vi "Get Firmware Version Names.vi"(8 "Error In":errorcluster, 9 "Device ID":u8, 11 "Device Family":T1) -> (0 "Error Out":errorcluster, 2 "Firmware Version Relative Path":string[](array[string]), 3 "Firmware Version Names":string[](array[string]))   [LabVIEW 2013, in "LVH-LINX.lvlib"]
doc: "Get Firmware Version Names for user specified Device Famile and Device ID."
uses:
  <vilib>/LabVIEW Hacker/LINX/LVH-LINX.lvlib
  <vilib>/LabVIEW Hacker/LINX/Private/Type Defs/Device Family.ctl
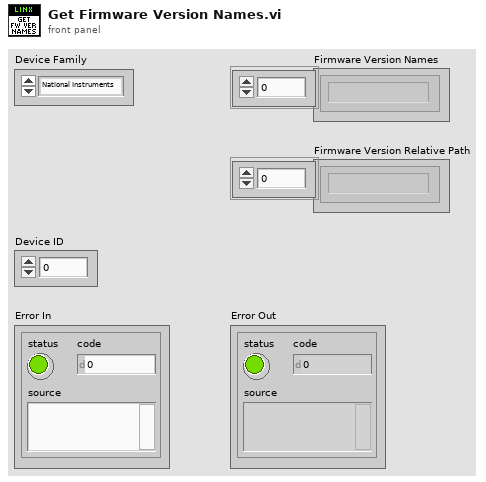
[diagram p1: front panel]
types:
  T1 = typedef "LVH-LINX.lvlib/Device Family.ctl" = enum8{"National Instruments", "Digilent", "Arduino"}
  T2 = typedef "LVH-LINX.lvlib/Generic Device.ctl" = cluster{"DI Channels":u8[], "DO Channels":u8[], "AI":u8[], "AO":u8[], "PWM":u8[], "QE":u8[], "UART":u8[], "I2C 2":u8[], "SPI":u8[], "CAN":u8[], "AI Ref (V)":dbl, "Firmware Program Interfaces":enum16{"N/A", "Serial / USB", "USB", "TCP"}[], "Firmware Versions":T3[], "Name":string, "AO Resolution (Bits)":u8, "AO Ref (V)":dbl}
  T3 = typedef "LVH-LINX.lvlib/Firmware Version.ctl" = cluster{"Name":string, "Relative Path":string, "Firmware Interface":T4}
  T4 = typedef "LVH-LINX.lvlib/Firmware Interface.ctl" = enum32{"Serial ", "Ethernet", "WIFI"}
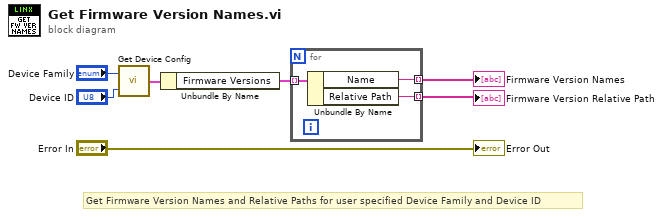
[diagram p0: block diagram]
diagram:
  # "Get Firmware Version Names and Relative Paths for user specified Device Family and Device ID"
  n1 = call <vilib>:"Get Device Config.vi"("Device ID"="Device ID", "Device Family"="Device Family") -> ("Device Config"=w7:T2)
  n2 = Unbundle By Name(w7) -> ("Firmware Versions"=w4:T3[])
  n3 = for {
    tunnel: w4 -> [w10] mode=indexing
    tunnel: [w9] -> w3 mode=indexing
    tunnel: [w8] -> w1 mode=indexing
    n4 = Unbundle By Name(w10) -> ("Name"=w9:string, "Relative Path"=w8:string)
  }
  "Firmware Version Names" <- w3
  "Firmware Version Relative Path" <- w1
  "Error Out" <- "Error In"
